vi "Export podataka.vi"() -> ()   [LabVIEW 2016]
uses:
  <vilib>/Waveform/WDTOps.llb/WDT Index Channel DBL.vi
  <vilib>/Waveform/WDTFileIO.llb/Export Waveforms To Spreadsheet File (1D).vi
panel:
  out "ACC 1":waveform(dbl)[](graph) caption="Signals"
  in  "ACC 2z":i32=5
  in  "ACC 2y":i32=4
  in  "ACC 2x":i32=3
  out "ACC 2":waveform(dbl)[](graph) caption="Signals"
  in  "ACC 1z":i32=2
  in  "ACC 1y":i32=1
  in  "ACC 1x":i32
  out "Ukupan Signal":dynamicdata(graph) caption="Signals"
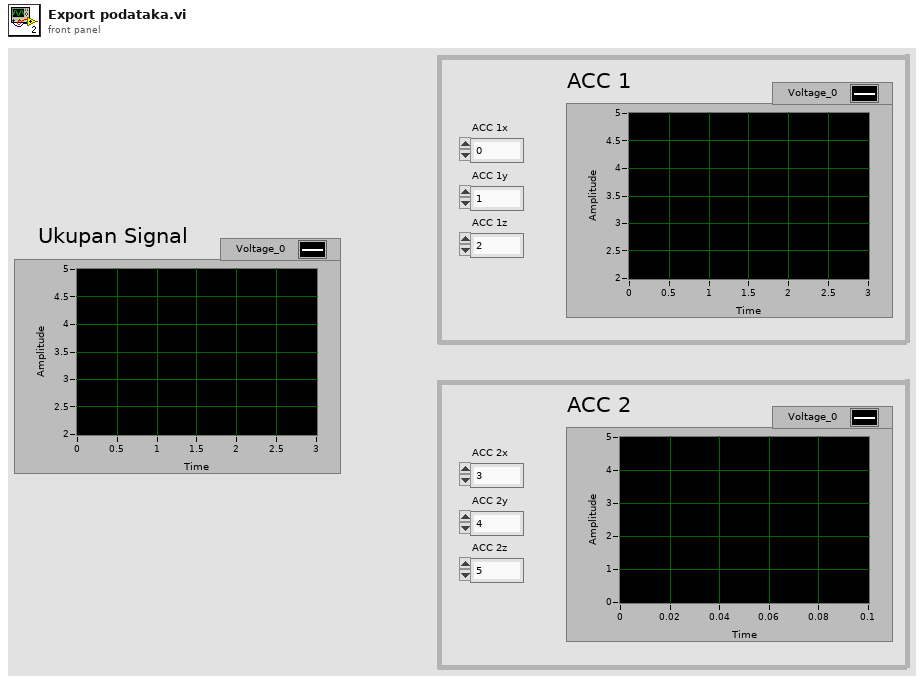
[diagram p1: front panel]
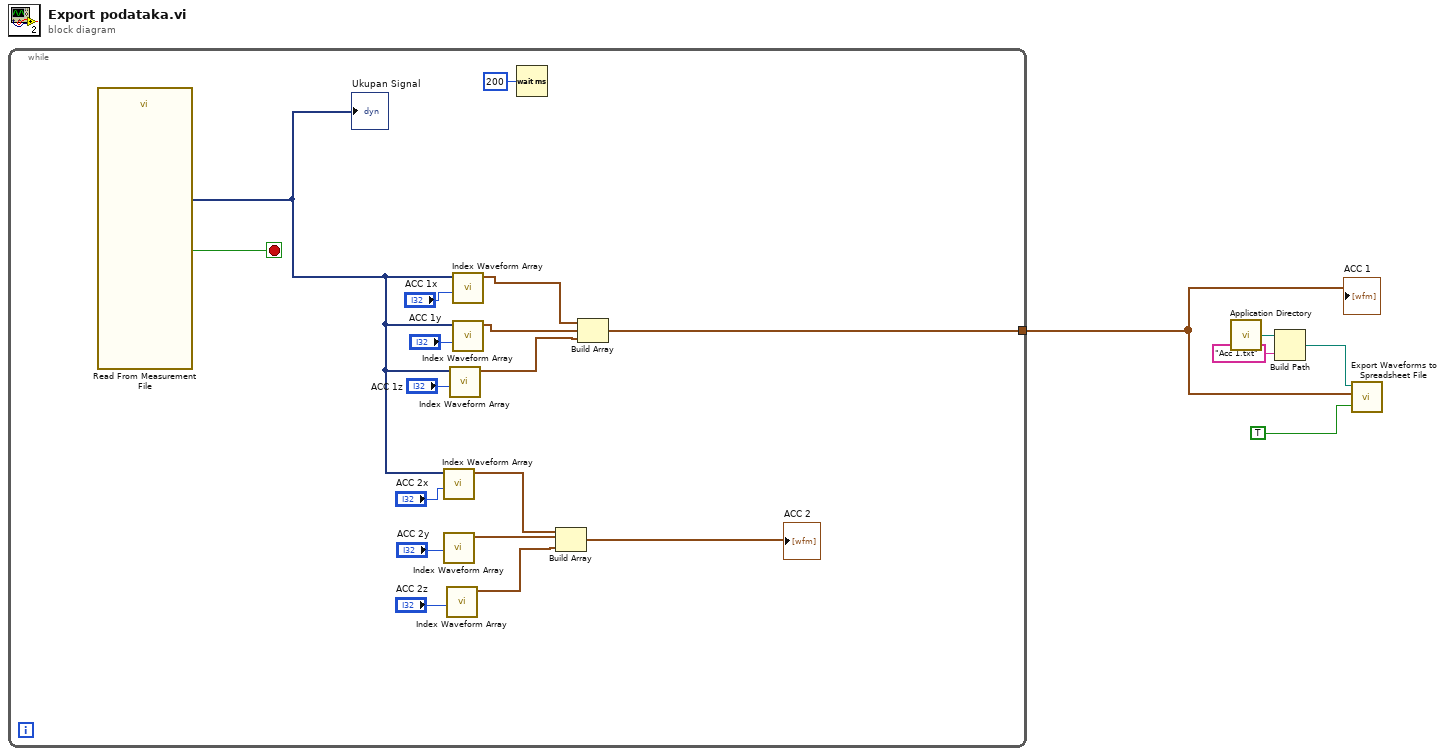
[diagram p0: block diagram]
diagram:
  n1 = while {
    tunnel: [w6] -> w1
    stop <- w21 stop-if-true
    n2 = call "Read From Measurement File"() -> ("Signals"=w17:dynamicdata, "EOF?"=w21:bool)  [unwired: 6 in, 4 out]
    "Ukupan Signal" <- w17
    n3 = call-poly <vilib>:"Index Waveform Array.vi"("index"="ACC 2x", "waveform array"=w17) -> ("waveform"=w10:waveform(dbl))  [unwired: 8 in, 1 out]
    n4 = call-poly <vilib>:"Index Waveform Array.vi"("index"="ACC 2y") -> ("waveform"=w9:waveform(dbl))  [unwired: 9 in, 1 out]
    n5 = call-poly <vilib>:"Index Waveform Array.vi"("index"="ACC 2z") -> ("waveform"=w8:waveform(dbl))  [unwired: 9 in, 1 out]
    n6 = call-poly <vilib>:"Index Waveform Array.vi"("index"="ACC 1z", "waveform array"=w17) -> ("waveform"=w18:waveform(dbl))  [unwired: 8 in, 1 out]
    n7 = call-poly <vilib>:"Index Waveform Array.vi"("index"="ACC 1x", "waveform array"=w17) -> ("waveform"=w20:waveform(dbl))  [unwired: 8 in, 1 out]
    n8 = call-poly <vilib>:"Index Waveform Array.vi"("index"="ACC 1y", "waveform array"=w17) -> ("waveform"=w19:waveform(dbl))  [unwired: 8 in, 1 out]
    n9 = Wait (ms)(milliseconds to wait=u32 200) -> ()  [unwired: 1 out]
    n10 = Build Array(w10, w9, w8) -> (→"ACC 2":waveform(dbl)[])
    n11 = Build Array(w20, w19, w18) -> (w6:waveform(dbl)[])
  }
  "ACC 1" <- w1
  n12 = call <vilib>:"Application Directory.vi"() -> ("Application Directory"=w4:path)
  n13 = Build Path(base path=w4, name or relative path="Acc 1.txt") -> (appended path=w2:path)
  n14 = call-poly <vilib>:"Export Waveforms to Spreadsheet File.vi"("append to file? (new file:F)"=TRUE, "waveforms"=w1, "file path (dialog if empty)"=w2) -> ()  [unwired: 7 in, 2 out]
